vi "test sppf.vi"() -> ()   [LabVIEW 2010]
panel:
  out "green rate":dbl format="%#_6p"
  out "ratio":dbl
  out "red rate":dbl format="%#_6p"
  out "theta out":dbl[](array[numeric])
  out "SPPF state out":T1
  in  "SPPF state":T1={"theta"=[0.0, 0.0], "w"=[[0.0, 0.0], [0.0, 0.0]], "elapsed time"=0.0}
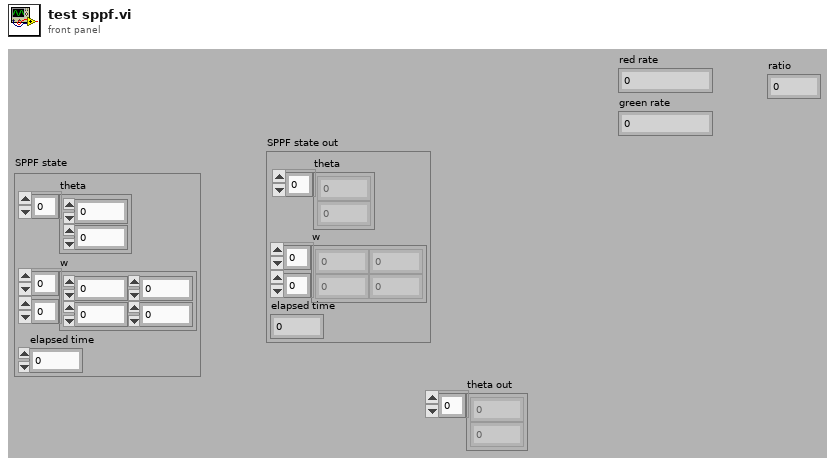
[diagram p1: front panel]
types:
  T1 = cluster{"theta":dbl[], "w":dbl[][], "elapsed time":dbl}
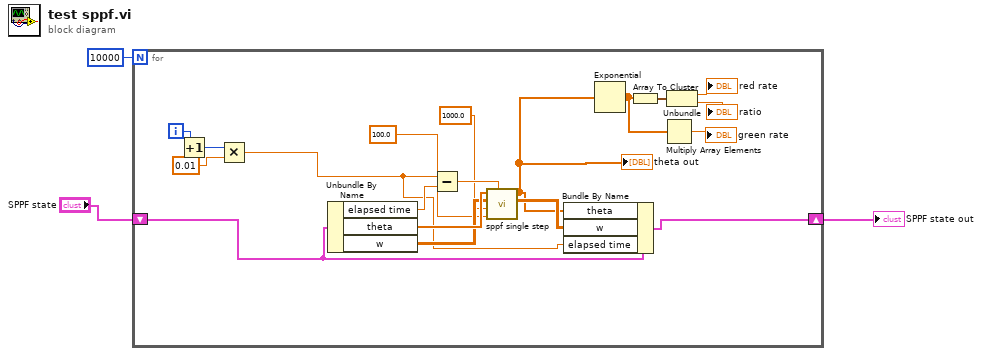
[diagram p0: block diagram]
diagram:
  n1 = for {
    N: 10000 -> [_]
    shift-right: [w5] -> w1
    shift-left: "SPPF state" -> [w6]
    i -> [w19]
    n2 = Increment(x=w19) -> (x+1=w4:i32)
    n3 = Multiply(x=w4, y=0.01) -> (x*y=w16:dbl)
    n4 = Unbundle By Name(w6) -> ("elapsed time"=w17:dbl, "theta"=w22:dbl[], "w"=w21:dbl[][])
    n5 = Subtract(x=w16, y=w17) -> (x-y=w15:dbl)
    n6 = call "sppf single step.vi"("dt"=w15, "num green photons"=100.0, "num red photons"=1000.0, "w"=w21, "theta"=w22) -> ("w"=w20:dbl[][], "theta"=w7:dbl[])  [unwired: 4 in, 1 out]
    "theta out" <- w7
    n7 = Bundle By Name(cluster=w6, "theta"=w7, "w"=w20, "elapsed time"=w16) -> (w5:T1)
    n8 = Exponential(1:w7) -> (0:w9:dbl[])
    n9 = Array To Cluster(array=w9) -> (cluster=w12:cluster{"[0]":dbl, "[1]":dbl})
    n10 = Multiply Array Elements(1:w9) -> (0:→"green rate":dbl)
    n11 = Unbundle(w12) -> ("[0]"=→"red rate":dbl, "[1]"=→"ratio":dbl)
  }
  "SPPF state out" <- w1
